vi "Write Model.lvclass.vi"(8 "error in (no error)":errorcluster, 10 "UserManagement.lvlib:Model":refnum<class "Model.lvclass">, 11 "PluginWithDatabase in":refnum<class "PluginWithDatabase.lvclass">) -> (0 "error out":errorcluster, 3 "PluginWithDatabase out":refnum<class "PluginWithDatabase.lvclass">)   [LabVIEW 2015, in "ActorManagement.lvlib" / "PluginWithDatabase.lvclass"]
uses:
  PluginWithDatabase.lvclass
  UserManagement/Model/Model.lvclass
  PluginWithDatabase.lvclass/PluginWithDatabase.ctl
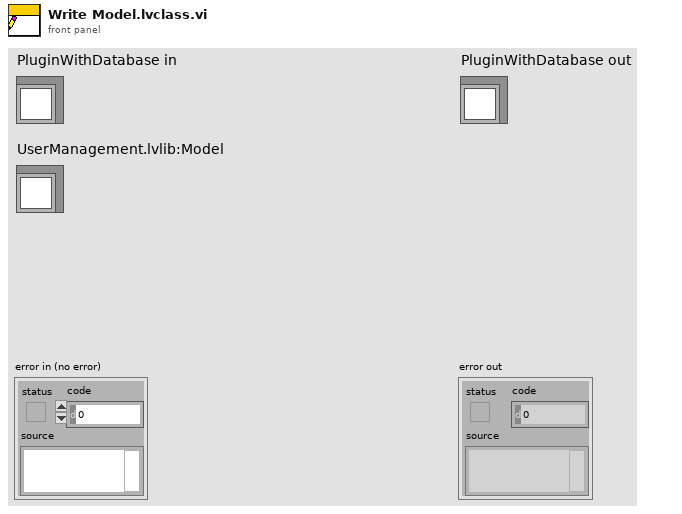
[diagram p1: front panel]
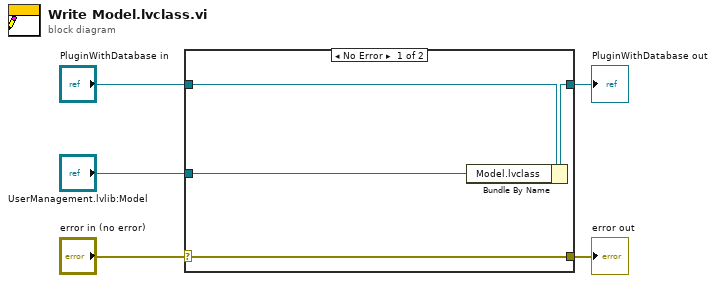
[diagram p0: block diagram]
diagram:
  n1 = case shown="No Error" "error in (no error)" {
    selector: "error in (no error)" -> [w9 w10]
    tunnel: [w9 w10] -> w4
    tunnel: [w7 w11] -> w2
    tunnel: "PluginWithDatabase in" -> [w8 w11]
    tunnel: "UserManagement.lvlib:Model" -> [w6 _]
    frame No Error {
      n2 = Bundle By Name(cluster=w8, "Model.lvclass"=w6) -> (w7:refnum<class "PluginWithDatabase.lvclass">)
    }
    frame Error {
    }
  }
  "error out" <- w4
  "PluginWithDatabase out" <- w2
